vi "r_from_pops.vi"(9 "rho- in":dbl[](array[numeric]), 10 "rho0 in":dbl[](array[numeric]), 11 "rho+ in":dbl[](array[numeric])) -> (3 "r array out":dbl[](array[numeric]))   [LabVIEW 2018]
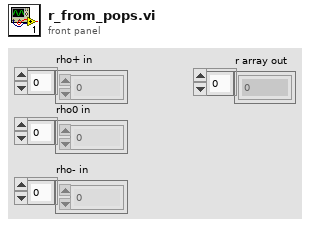
[diagram p1: front panel]
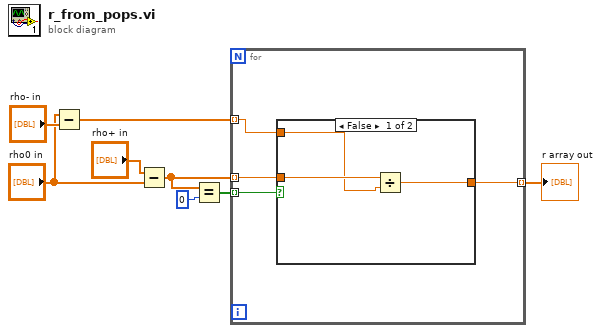
[diagram p0: block diagram]
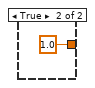
[diagram p2: hidden frame]
diagram:
  n1 = Subtract(x="rho0 in", y="rho- in") -> (x-y=w5:dbl[])
  n2 = Subtract(x="rho+ in", y="rho0 in") -> (x-y=w4:dbl[])
  n3 = Equal?(x=w4, y=0) -> (x = y?=w2:bool[])
  n4 = for {
    tunnel: w4 -> [w12] mode=indexing
    tunnel: w5 -> [w9] mode=indexing
    tunnel: [w11] -> w1 mode=indexing
    tunnel: w2 -> [w10] mode=indexing
    n5 = case shown="False" w10 {
      tunnel: w12 -> [w14 _]
      tunnel: [w15 1.0] -> w11
      tunnel: w9 -> [w13 _]
      frame False {
        n6 = Divide(x=w14, y=w13) -> (x/y=w15:dbl)
      }
      frame True {
      }
    }
  }
  "r array out" <- w1
